vi "tableToJson.vi"(1 "data":string[](array[string])) -> (0 "json":string)   [LabVIEW 2019]
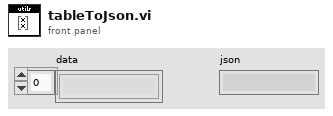
[diagram p1: front panel]
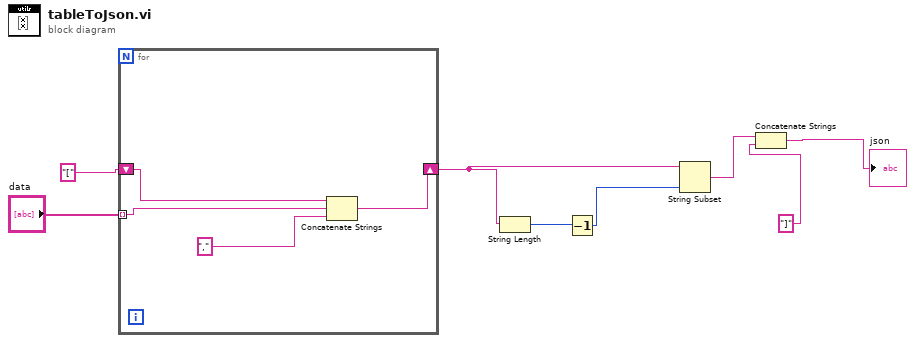
[diagram p0: block diagram]
diagram:
  n1 = for {
    tunnel: "data" -> [w10] mode=indexing
    shift-right: [w12] -> w2
    shift-left: "[" -> [w11]
    n2 = Concatenate Strings(w11, w10, "," ("string")) -> (w12:string)
  }
  n3 = String Length(string=w2) -> (length=w3:i32)
  n4 = Decrement(x=w3) -> (x-1=w5:i32)
  n5 = String Subset(string=w2, length (rest)=w5) -> (substring=w4:string)  [unwired: 1 in]
  n6 = Concatenate Strings(w4, "]" ("string")) -> (→"json":string)
